vi "Launcher.vi"() -> ()   [LabVIEW 2020]
uses:
  UI Actor/UI Actor.lvclass
  C:/Program Files (x86)/National Instruments/LabVIEW 2020/vi.lib/ActorFramework/Actor/Actor.lvclass
  UI Actor/UI Actor.lvclass/UI Actor.ctl
  UI Actor/Write Coins.vi
  UI Actor/Write Products.vi
  <vilib>/ActorFramework/Actor/Actor.lvclass
panel:
  in  "Products":enum16{"COCA", "NEStle"}(ring)
  in  "Coins":enum16{"MXN", "USD"}(ring)
  # "Seleccione el tipo de moneada"
  # "Seleccione el tipo de producto"
  # "Bienvenido a la\nmaquina \nExpndedora\n\n\nMEZA TECHNOLOGY"
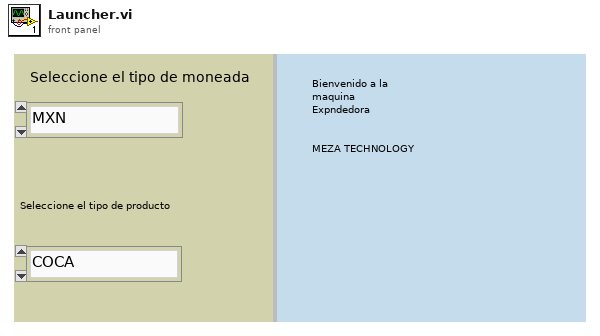
[diagram p1: front panel]
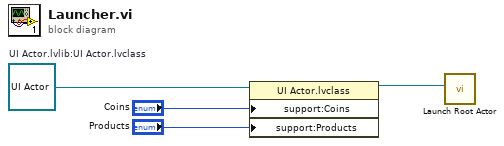
[diagram p0: block diagram]
diagram:
  w4 = refnum<class "UI Actor.lvclass"> refnum  # UI Actor.lvlib:UI Actor.lvclass
  n1 = property class="UI Actor.lvclass"(reference=w4, "support:Coins"="Coins", "support:Products"="Products") -> (reference out=w3:refnum<class "UI Actor.lvclass">)  [unwired: 1 in, 1 out]
  n2 = call <vilib>:"Launch Root Actor.vi"("Actor"=w3) -> ()  [unwired: 9 in, 2 out]
